vi "Initialize Daemon.vi"(8 "error in":errorcluster, 9 "Data Model":refnum<class "Device Data Model.lvclass">, 10 "transmission data unit":refnum<class "Transmission Data Unit.lvclass">, 11 "Serial Slave in":refnum<class "Serial Slave.lvclass">) -> (0 "error out":errorcluster, 3 "Serial Slave out":refnum<class "Serial Slave.lvclass">)   [LabVIEW 2012, in "Serial Slave.lvclass"]
doc: "This provides an interface for the slave to launch a protocol daemon."
uses:
  Serial Slave.lvclass
  Transmission Data Unit/Transmission Data Unit.lvclass
  Data Model/Device Data Model.lvclass
  Transmission Data Unit/Serial Interface/Serial Data Unit.lvclass
  Serial Slave.lvclass/Serial Slave.ctl
  Transmission Data Unit/Transmission Data Unit.lvclass/Transmission Data Unit.ctl
  Network Slave.lvclass
  Read VISA resource name.vi
  Read Baud Rate.vi
  Read Parity.vi
  Read Flow Control.vi
  Serial Daemon.vi
  Serial Shared Components/Serial Shared Components.lvlib
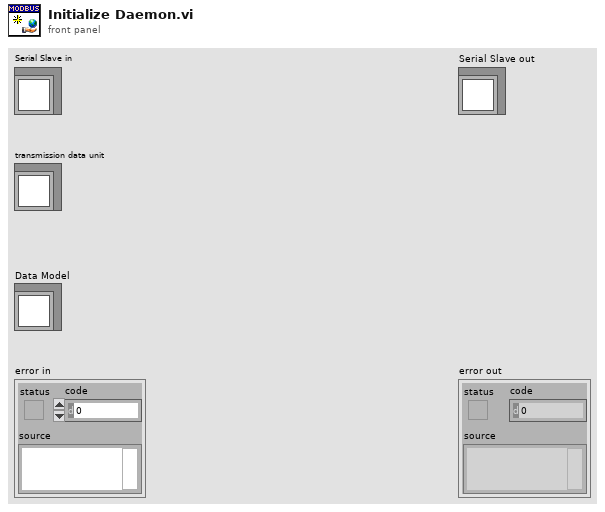
[diagram p1: front panel]
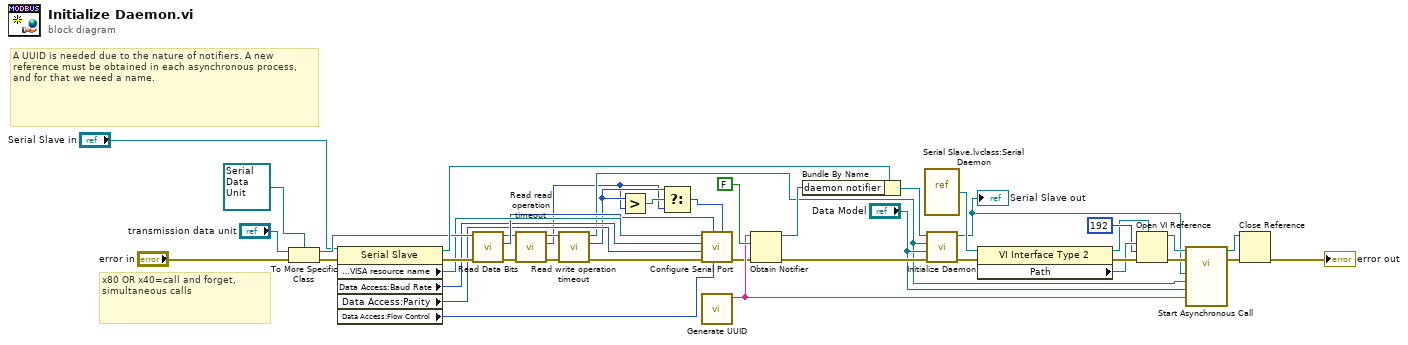
[diagram p0: block diagram]
diagram:
  # "x80 OR x40=call and forget, simultaneous calls"
  # "A UUID is needed due to the nature of notifiers. A new reference must be obtained in each asynchronous process, and for that we need a name."
  n1 = To More Specific Class(target class=refnum<class "Serial Data Unit.lvclass"> refnum ("Serial Data Unit in"), reference="transmission data unit", error in="error in") -> (specific class reference=w29:refnum<class "Serial Data Unit.lvclass">, error out=w31:errorcluster)
  n2 = property class="Serial Slave"(reference="Serial Slave in", error in=w31) -> (reference out=w33:refnum<class "Serial Slave.lvclass">, error out=w42:errorcluster, "Data Access:VISA resource name"=w27:refnum<visa-resource-name>, "Data Access:Baud Rate"=w25:u32, "Data Access:Parity"=w24:u16, "Data Access:Flow Control"=w23:u16)
  n3 = call-dynamic "Read Data Bits.vi"("error in (no error)"=w42, "Serial Data Unit in"=w29) -> ("error out"=w9:errorcluster, "data bits"=w26:u16, "Serial Data Unit out"=w12:refnum<class "Serial Data Unit.lvclass">)  [unwired: 7 in]
  n4 = call "Read read operation timeout.vi"("error in (no error)"=w9, "transmission data unit in"=w12) -> ("error out"=w10:errorcluster, "read operation timeout"=w6:i32, "transmission data unit out"=w13:refnum<class "Serial Data Unit.lvclass">)  [unwired: 7 in]
  n5 = call "Read write operation timeout.vi"("error in (no error)"=w10, "transmission data unit in"=w13) -> ("error out"=w4:errorcluster, "write operation timeout"=w7:i32, "transmission data unit out"=w11:refnum<class "Serial Data Unit.lvclass">)  [unwired: 7 in]
  n6 = Greater?(x=w7, y=w6) -> (0:w8:bool)
  n7 = Select(t=w7, s=w8, f=w6) -> (s? t:f=w5:i32)
  n8 = call "Configure Serial Port.vi"("Timeout"=w5, "Flow Control"=w23, "data bits"=w26, "error in (no error)"=w4, "Parity"=w24, "Baud Rate"=w25, "VISA Refnum in"=w27) -> ("error out"=w22:errorcluster)  [unwired: 4 in]
  n9 = call "Generate UUID.vi"() -> ("UUID"=w34:string)  [unwired: 11 in]
  n10 = Obtain Notifier(name (unnamed)=w34, notification data type=FALSE, error in (no error)=w22) -> (notifier out=w35:refnum<notifier>, error out=w20:errorcluster)  [unwired: 1 in, 1 out]
  n11 = Bundle By Name(cluster=w33, "daemon notifier"=w35) -> (w17:refnum<class "Serial Slave.lvclass">)
  n12 = vi-ref "Serial Slave.lvclass:Serial Daemon.vi"() -> (w41:refnum<vi>)
  n13 = call-parent "Initialize Daemon.vi"("error in"=w20, "Data Model"="Data Model", "transmission data unit"=w11, "network slave in"=w17) -> ("error out"=w19:errorcluster, "network slave out"=w18:refnum<class "Serial Slave.lvclass">)  [unwired: 6 in]
  "Serial Slave out" <- w18
  n14 = property class="VI Interface Type 2"(reference=w41, error in=w19) -> (reference out=w2:refnum<vi>, error out=w40:errorcluster, "Path"=w39:path)
  n15 = Open VI Reference(type specifier VI Refnum (for type only)=w2, vi path=w39, options=192 ("x .or. y?"), error in (no error)=w40) -> (vi reference=w38:refnum<vi>, error out=w36:errorcluster)  [unwired: 2 in]
  n16 = call-by-ref "Start Asynchronous Call"(reference=w38, error in=w36, "UUID"=w34, "Data Model"="Data Model", "transmission data unit"=w11, "serial slave"=w18) -> (reference out=w3:refnum<vi>, error out=w28:errorcluster)  [unwired: 8 in]
  n17 = Close Reference(reference=w3, error in (no error)=w28) -> (error out=→"error out":errorcluster)
